vi "Insert Reserved Error.vi"(4 "error in (no error)":errorcluster, 5 "non-standard source (\"\")":string, 6 "Reserved Error Code":u16(ring) items=["No error", "Argument error", "Memory is full", "Out of zone", "End of file", "File already open", "Generic file I/O error", "File not found", "File permission error", "Disk is full", "Duplicate path", "Too many files open", "System feature not enabled", "Resource file not found", "Cannot add resource", "Resource not found", "Image not found", "Image memory error", "Pen does not exist", "Config type invalid", "Config token not found", "Config parse error", "Config memory error", "Bad external code format", "Bad external code offset", "External code not present", "Null window", "Destroy window error", "Null menu", "Print aborted", "Bad print record", "Print driver error", "Windows error during printing", "Memory error during printing", "Print dialog error", "Generic print error", "Invalid device refnum", "Device not found", "Device parameter error", "Device unit error", "Cannot open device", "Device call aborted", "Generic error", "Cancelled by user", "Object ID too low", "Object ID too high", "Object not in heap", "Unknown heap", "Unknown object (invalid DefProc)", "Unknown object (DefProc not in table)", "Message out of range", "Invalid (null) method", "Unknown message", "Manager call not supported", "Bad address", "Network operation in progress", "Network operation timed out", "Connection is busy", "Network attribute not supported", "Network error", "Address in use", "System out of memory", "Connection aborted", "Connection refused", "Not connected", "Already connected", "Connection closed", "Initialization error (interapplication manager)", "Bad occurrence", "Wait on unbound occurrence handler", "Occurrence queue overflow", "Datalog type conflict", "Unused", "Unrecognized type (interapplication manager)", "Memory corrupt", "Failed to make temporary DLL", "Old CIN version", "Drag socket not found", "Failed to load drop-object", "Failed to register OLE object", "Failed to release OLE object", "Format specifier type mismatch", "Unknown format specifier", "Too few format specifiers", "Too many format specifiers", "Scan failed", "Newer CIN version", "OLE Convert", "Runtime menu error", "Password tampered", "Unknown error code"], 7 "error? (True)":bool=TRUE) -> (0 "error out":errorcluster)   [LabVIEW 2015]
doc: "Wire \"Reserved error code\" with an error ring constant to be inserted unless there's an upstream error or \"error?\" is false. Source string is built from the calling chain, starting with this vi's caller, unless the \"non-standard source\" input is wired.\n\nFreeware from Moore Good Ideas, www.mooregoodideas.com. Do not remove this line."
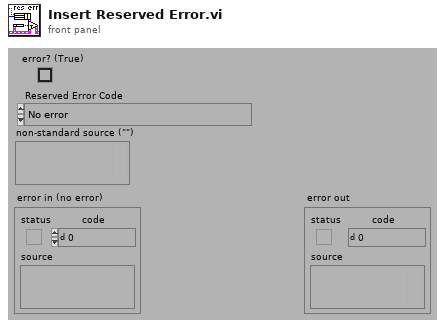
[diagram p1: front panel]
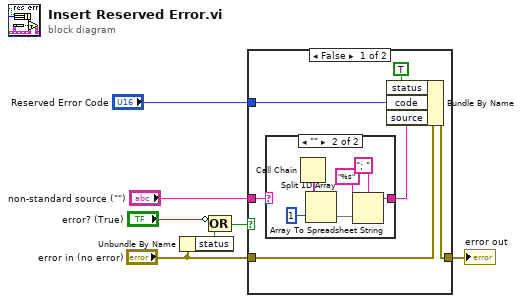
[diagram p0: block diagram]
diagram:
  n1 = Unbundle By Name("error in (no error)") -> ("status"=w2:bool)
  n2 = Compound Arithmetic op=OR(invert "error? (True)", w2) -> (w1:bool)
  n3 = case shown="False" w1 {
    tunnel: "error in (no error)" -> [w12 w21]
    tunnel: [w9 w21] -> w5
    tunnel: "non-standard source (\"\")" -> [w13 _]
    tunnel: "Reserved Error Code" -> [w8 _]
    frame False {
      n4 = case shown="\"\"" w13 {
        selector: w13 -> [w14 _]
        tunnel: [w14 w15] -> w11
        frame Default {
        }
        frame "" {
          n5 = Call Chain() -> (call chain=w19:string[])
          n6 = Split 1D Array(array=w19, index=1) -> (second subarray=w17:string[])  [unwired: 1 out]
          n7 = Array To Spreadsheet String(delimiter (Tab)="; ", array=w17, 3:"%s" ("format string")) -> (spreadsheet string=w15:string)
        }
      }
      n8 = Bundle By Name(cluster=w12, "status"=TRUE ("Bundle Element"), "code"=w8, "source"=w11) -> (w9:errorcluster)
    }
    frame True {
    }
  }
  "error out" <- w5
